vi "ActiveObjects_DynamicEvents_ControlWindow_5x6x5.vi"(0 "reference in":refnum<class>, 5 "ShowProcessWindow":bool, 11 "Error In":errorcluster) -> (4 "reference out":refnum<class>, 15 "Error Out":errorcluster)   [LabVIEW 2020]
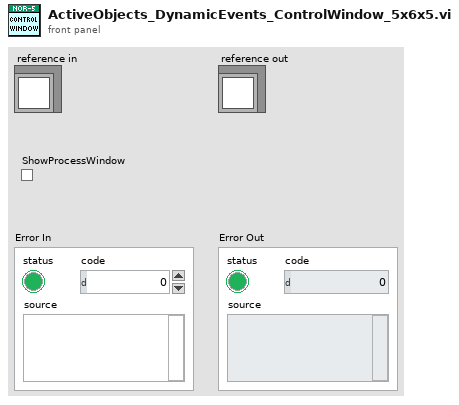
[diagram p1: front panel]
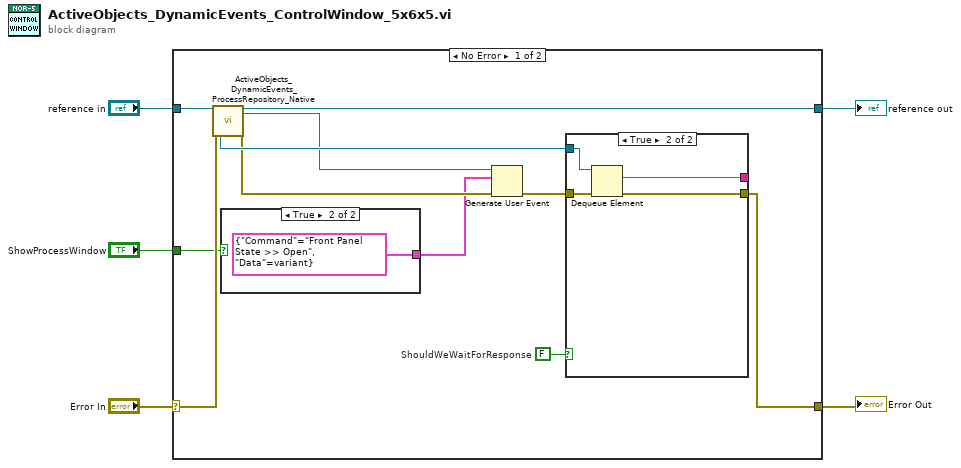
[diagram p0: block diagram]
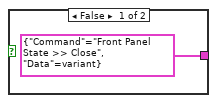
[diagram p2: hidden frame]
diagram:
  n1 = case shown="No Error" "Error In" {
    selector: "Error In" -> [w16 w25]
    tunnel: [w8 w25] -> w4
    tunnel: [w14 w24] -> w2
    tunnel: "reference in" -> [w15 w24]
    tunnel: "ShowProcessWindow" -> [w6 _]
    frame No Error {
      w13 = FALSE  # ShouldWeWaitForResponse
      n2 = call "ActiveObjects_DynamicEvents_ProcessRepository_Native.vi"("reference in"=w15, "Error In"=w16) -> ("QueueFromProcess"=w11:refnum<queue>, "reference out"=w14:refnum<class>, "EventsToProcess"=w9:refnum<user-event>, "Error Out"=w10:errorcluster)  [unwired: 10 in, 4 out]
      n3 = case shown="True" w6 {
        tunnel: [cluster{"Command":string, "Data":variant} {"Command"="Front Panel State >> Close", "Data"=variant} ("MessageToProcess") cluster{"Command":string, "Data":variant} {"Command"="Front Panel State >> Open", "Data"=variant} ("MessageToProcess")] -> w7
        frame False {
        }
        frame True {
        }
      }
      n4 = Generate User Event(user event=w9, event data cluster=w7, error in=w10) -> (error out=w12:errorcluster)  [unwired: 1 in, 1 out]
      n5 = case shown="True" w13 {
        tunnel: w12 -> [w19 w23]
        tunnel: w11 -> [_ w22]
        tunnel: [_ w21] -> _
        tunnel: [w19 w20] -> w8
        frame False {
        }
        frame True {
          n6 = Dequeue Element(queue=w22, error in (no error)=w23) -> (element=w21:string, error out=w20:errorcluster)  [unwired: 1 in, 2 out]
        }
      }
    }
    frame Error {
    }
  }
  "Error Out" <- w4
  "reference out" <- w2
